vi "Get True Solar Time.vi"(6 "Eq of Time (min)":dbl, 10 "time (utc)":timestamp format="%<%H:%M:%S\n%x>T", 11 "Long":dbl) -> (3 "TST (min)":dbl)   [LabVIEW 2014, in "Solar Calculations.lvlib"]
uses:
  Solar Calculations.lvlib
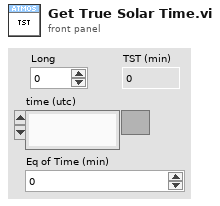
[diagram p1: front panel]
types:
  T1 = typedef "LVDateTimeRec.ctl" = cluster{"fractional second":dbl, "second":i32, "minute":i32, "hour":i32, "day of month":i32, "month":i32, "year":i32, "day of week":i32, "day of year":i32, "DST":i32}
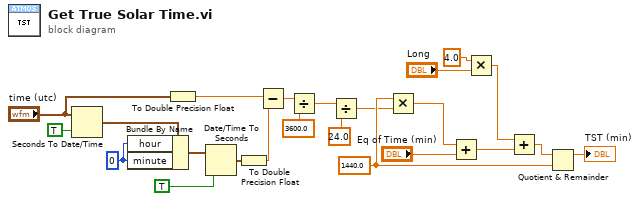
[diagram p0: block diagram]
diagram:
  w14 = 0 ("minute")
  w22 = 1440.0 ("x")
  n1 = Seconds To Date/Time(time stamp (now)="time (utc)", to UTC (F)=TRUE) -> (date time rec=w4:T1)
  n2 = Bundle By Name(cluster=w4, "hour"=w14, "minute"=w14) -> (w13:T1)
  n3 = To Double Precision Float(number="time (utc)") -> (double precision float=w1:dbl)
  n4 = Date/Time To Seconds(1:TRUE ("is UTC (F)"), 2:w13) -> (0:w8:timestamp)
  n5 = To Double Precision Float(number=w8) -> (double precision float=w7:dbl)
  n6 = Subtract(x=w1, y=w7) -> (x-y=w12:dbl)
  n7 = Divide(x=w12, y=3600.0) -> (x/y=w10:dbl)
  n8 = Divide(x=w10, y=24.0) -> (x/y=w3:dbl)
  n9 = Multiply(x=w22, y=w3) -> (x*y=w16:dbl)
  n10 = Add(x=w16, y="Eq of Time (min)") -> (x+y=w19:dbl)
  n11 = Multiply(x=4.0 ("y"), y="Long") -> (x*y=w20:dbl)
  n12 = Add(x=w20, y=w19) -> (x+y=w21:dbl)
  n13 = Quotient & Remainder(x=w21, y=w22) -> (x-y*floor(x/y)=→"TST (min)":dbl)  [unwired: 1 out]
